vi "Find_Top_Target.vi"(8 "Difference Image":T1, 11 "Particle Reports (Pixels)":T3(array[cluster])) -> (2 "Found Target":bool, 3 "Top Target":T2)   [LabVIEW 2011]
uses:
  <vilib>/vision/Image Controls.llb/IMAQ Image.ctl
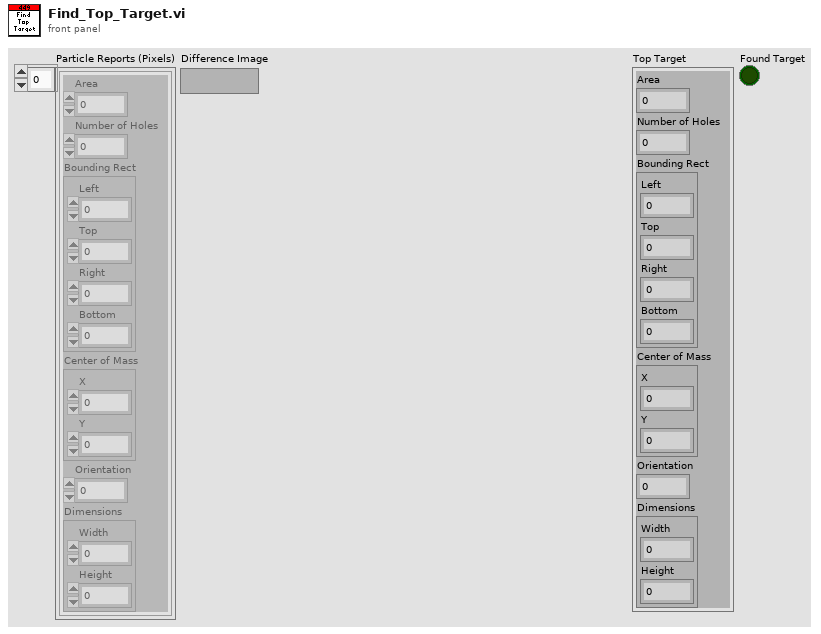
[diagram p1: front panel]
types:
  T1 = typedef "IMAQ Image.ctl" = refnum<image>
  T2 = cluster{"Area":dbl, "Number of Holes":dbl, "Bounding Rect":cluster{"Left":dbl, "Top":dbl, "Right":dbl, "Bottom":dbl}, "Center of Mass":cluster{"X":dbl, "Y":dbl}, "Orientation":dbl, "Dimensions":cluster{"Width":dbl, "Height":dbl}}
  T3 = cluster{"Area":dbl, "Number of Holes":dbl, "Bounding Rect":cluster{"Left":dbl, "Top":dbl, "Right":dbl, "Bottom":dbl}, "Center of Mass":cluster{"X":dbl, "Y":dbl}, "Orientation":dbl, "Dimensions":cluster{"Width":dbl, "Height":dbl}}[]
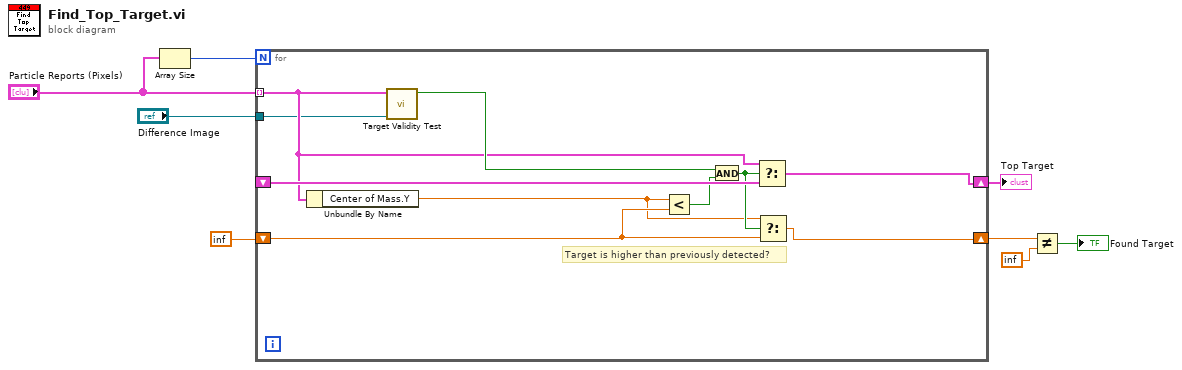
[diagram p0: block diagram]
diagram:
  n1 = Array Size(array="Particle Reports (Pixels)") -> (size(s)=w7:i32)
  n2 = for {
    N: w7 -> [_]
    tunnel: "Particle Reports (Pixels)" -> [w10] mode=indexing
    shift-right: [w13] -> w4
    shift-left: inf -> [w14]
    shift-right: [w16] -> w5
    shift-left: _ -> [w18]
    tunnel: "Difference Image" -> [w9]
    # "Target is higher than previously detected?"
    n3 = Unbundle By Name(w10) -> ("Center of Mass.Y"=w11:dbl)
    n4 = call "Target Validity Test.vi"("Difference Image"=w9, "Particle Report"=w10) -> ("Target is valid?"=w12:bool)  [unwired: 9 in]
    n5 = Less?(x=w11, y=w14) -> (x < y?=w17:bool)
    n6 = And(x=w12, y=w17) -> (x .and. y?=w15:bool)
    n7 = Select(t=w10, s=w15, f=w18) -> (s? t:f=w16:T2)
    n8 = Select(t=w11, s=w15, f=w14) -> (s? t:f=w13:dbl)
  }
  "Top Target" <- w5
  n9 = Not Equal?(x=w4, y=inf) -> (x != y?=→"Found Target":bool)
